vi "OSU_Get_Device_ID.vi"(8 "error in (no error)":errorcluster) -> (0 "error out":errorcluster, 1 "id":string[](array[string]), 3 "Reference out":refnum<k24>)   [LabVIEW 2017]
uses:
  LV_IL_Sample/DLL/InstrumentDLL.dll
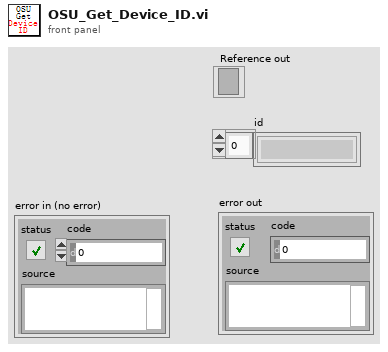
[diagram p1: front panel]
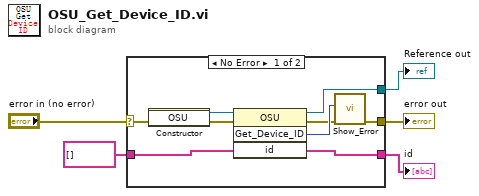
[diagram p0: block diagram]
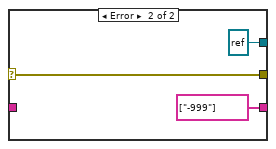
[diagram p2: hidden frame]
diagram:
  n1 = case shown="No Error" "error in (no error)" {
    selector: "error in (no error)" -> [w9 w17]
    tunnel: [w14 string[] ["-999"] ("id")] -> w5
    tunnel: string[] [] ("id") -> [w13 _]
    tunnel: [w10 refnum<k24> refnum ("new reference")] -> w3
    tunnel: [w6 w17] -> w2
    frame No Error {
      n2 = constructor class="OSU"(error in=w9) -> (reference out=w11:refnum<k24>, error out=w12:errorcluster)  [unwired: 2 in, 1 out]
      n3 = invoke on="调用节点" class="OSU" method="Get_Device_ID"(reference=w11, error in=w12, "id"=w13) -> (reference out=w10:refnum<k24>, error out=w7:errorcluster, "Get_Device_ID"=w8:i32, "id"=w14:string[])  [unwired: 1 in]
      n4 = call "Show_Error.vi"("error in (no error)"=w7, "Error"=w8) -> ("error out"=w6:errorcluster)  [unwired: 9 in]
    }
    frame Error {
    }
  }
  "id" <- w5
  "error out" <- w2
  "Reference out" <- w3
